vi "DBClient2.vi"() -> ()   [LabVIEW 2015]
uses:
  <vilib>/addons/database/Connection.llb/DB Tools Open Connec (Path).vi
  <vilib>/addons/database/Connection.llb/Conn Execute.vi
  <vilib>/addons/database/Recordset.llb/Rec Fetch Recordset Data (R).vi
  <vilib>/addons/database/Recordset.llb/Rec Destroy - Connection.vi
  <vilib>/addons/database/_DB Variant To Data/Database Variant To Data.xnode
  <vilib>/addons/database/NI_Database_API.lvlib
panel:
  in  "stop":bool
  out "Table link_buku_kategori":string[][](table)
  out "Table link_buku_pengarang":string[][](table)
  out "Table Buku":string[][](table)
  in  "Insert Button link_buku_kategori":bool
  in  "kategori_id lbk":string
  in  "buku_isbn lbk":string
  in  "Insert Button link_buku_pengarang":bool
  in  "pengarang_id lbp":string
  in  "buku_isbn lbp":string
  in  "buku_harga":string
  in  "buku_deskripsi":string
  in  "buku_jmlhalaman":string
  in  "buku_tgl_terbit":string
  in  "penerbit_id buku":string
  in  "buku_judul":string
  in  "buku_ISBN":string
  in  "Insert Button Buku":bool
  out "Table Penerbit":string[][](table)
  in  "Insert Button Penerbit":bool
  in  "Nama Penerbit":string
  in  "ID Penerbit":string
  out "Table Kategori":string[][](table)
  in  "Nama Kategori":string
  in  "ID Kategori":string
  in  "Insert Button Kategori":bool
  in  "Nama Pengarang":string
  in  "ID Pengarang":string
  in  "Insert Button Pengarang":bool
  out "Table Pengarang":string[][](table)
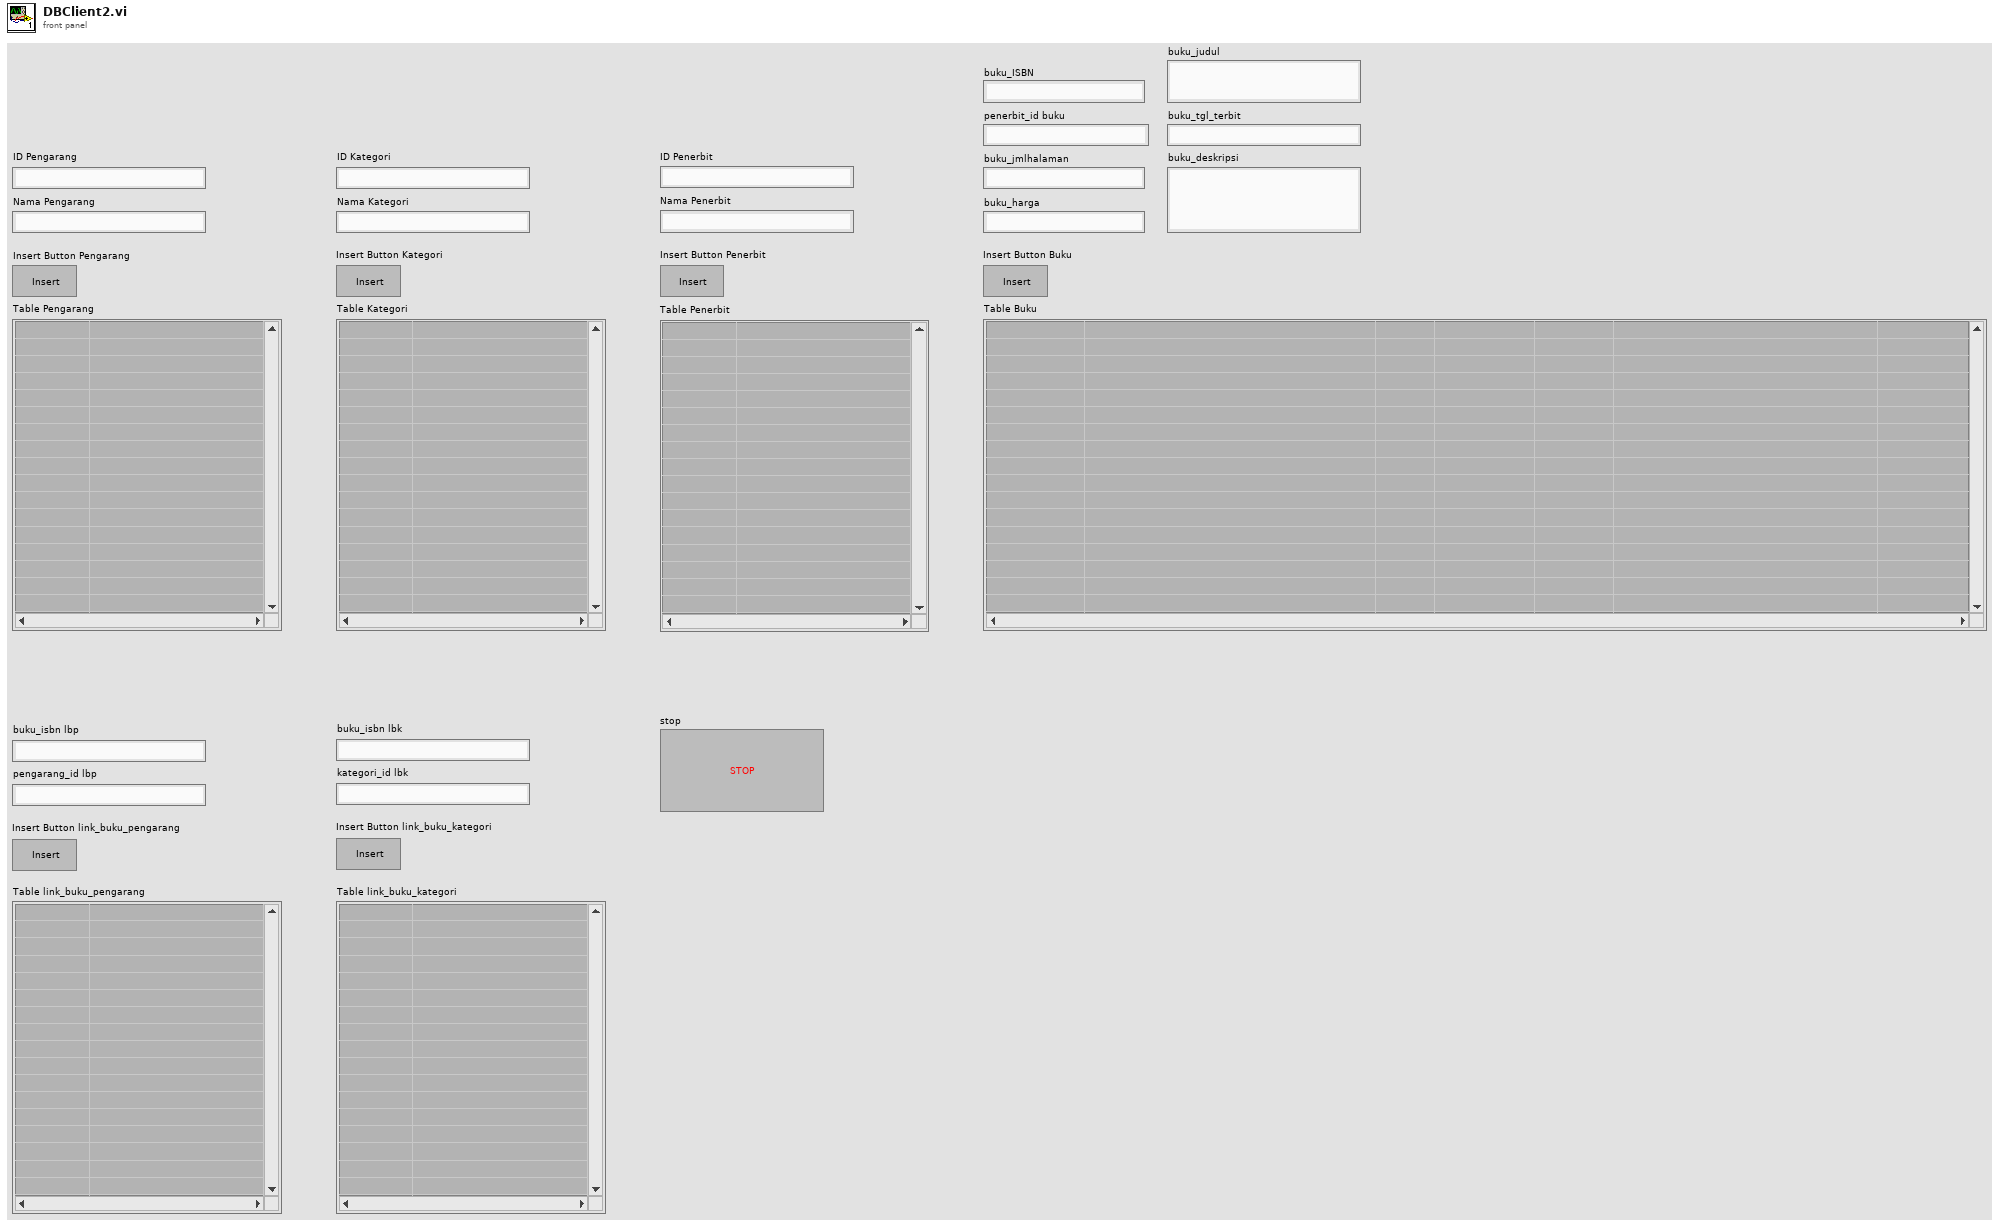
[diagram p1: front panel]
types:
  T1 = typedef "NI_Database_API.lvlib/Conn ObjectReference.ctl" = refnum<k1>
  T2 = typedef "NI_Database_API.lvlib/Rec ObjectReference.ctl" = refnum<k1>
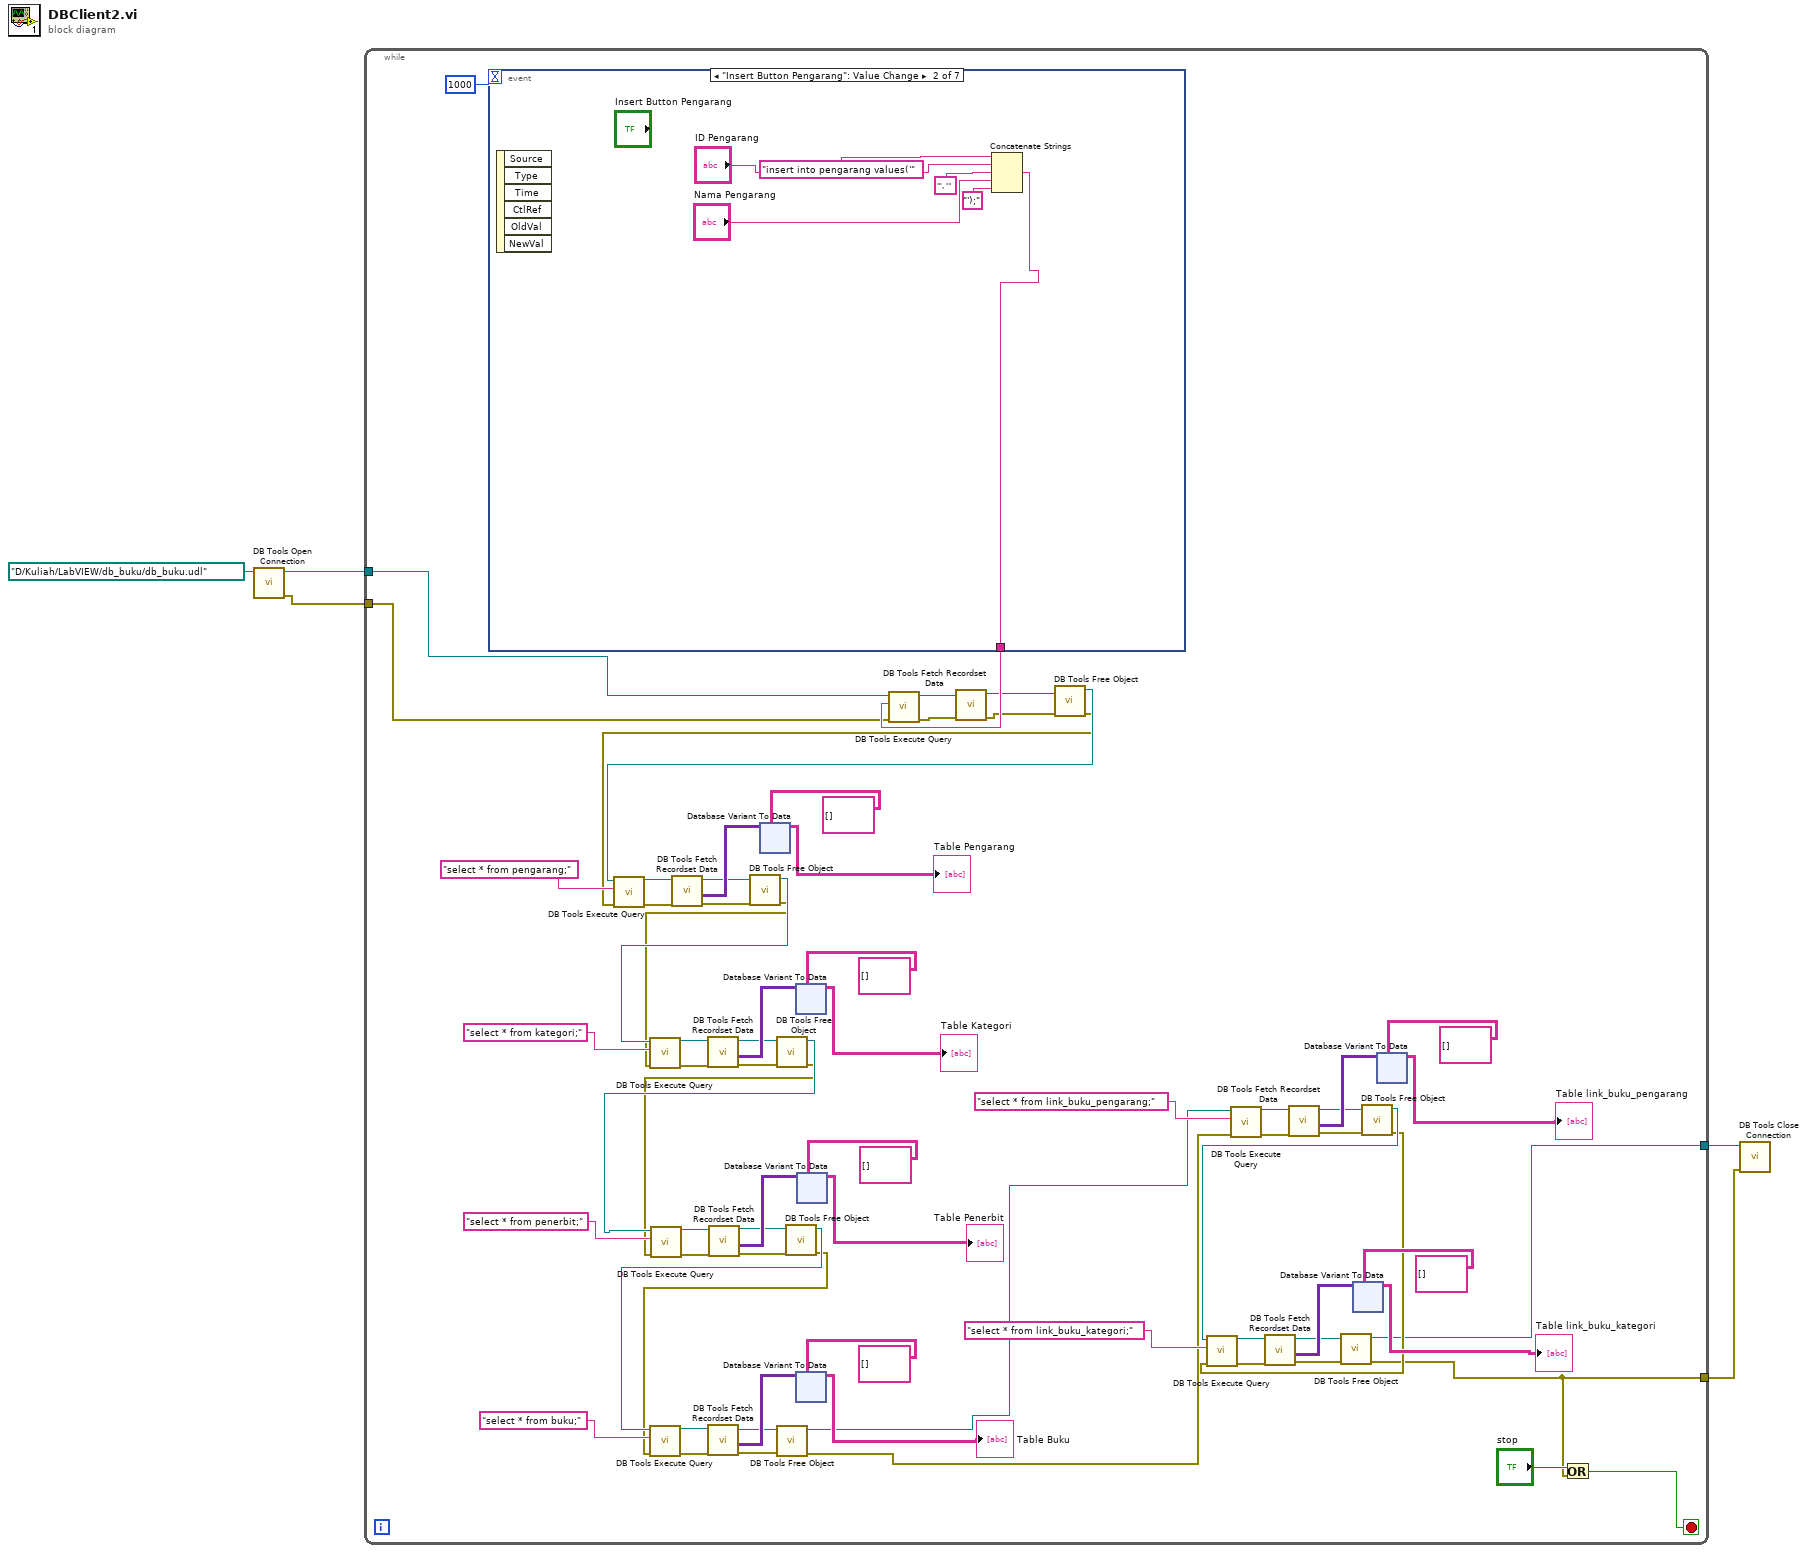
[diagram p0: block diagram]
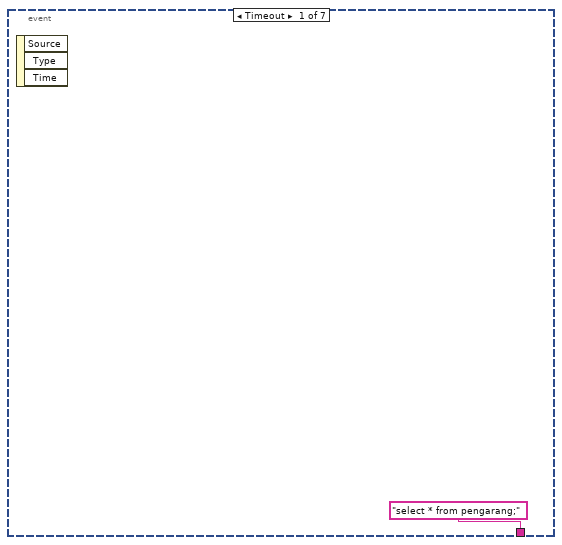
[diagram p2: hidden frame]
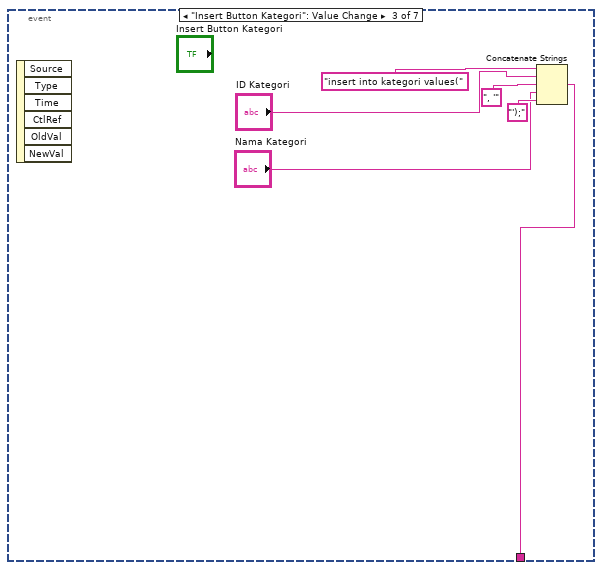
[diagram p3: hidden frame]
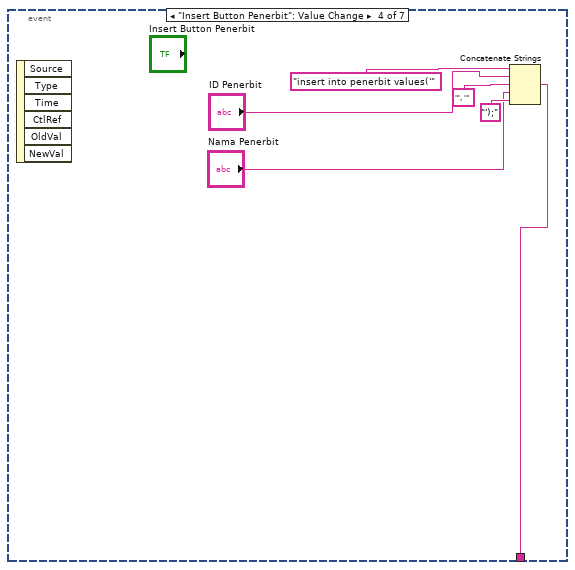
[diagram p4: hidden frame]
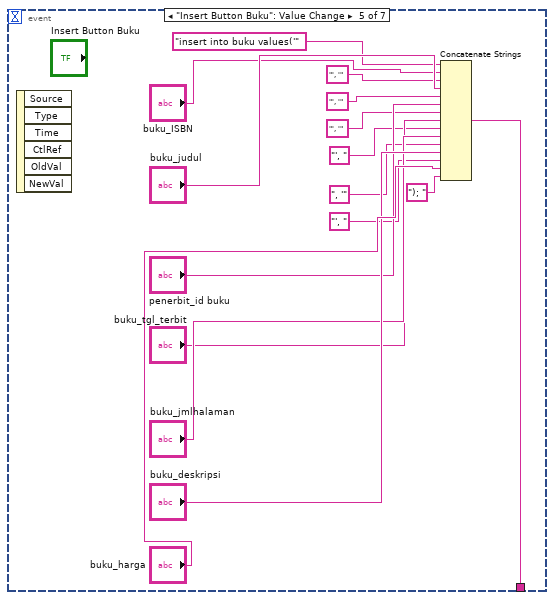
[diagram p5: hidden frame]
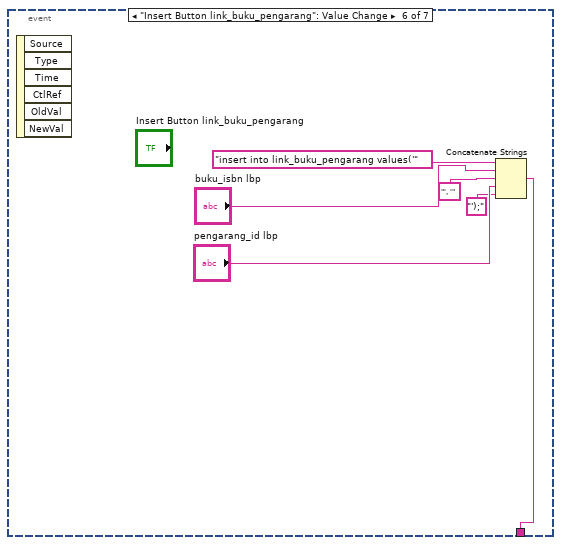
[diagram p6: hidden frame]
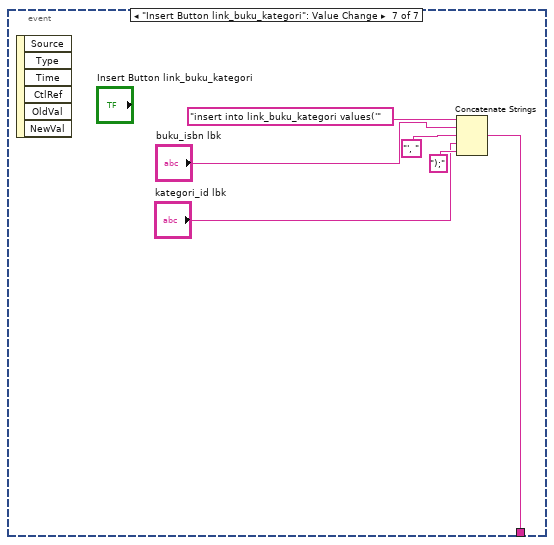
[diagram p7: hidden frame]
diagram:
  n1 = call-poly <vilib>:"DB Tools Open Connection.vi"("connection information"=path "D:/Kuliah/LabVIEW/db_buku/db_buku.udl") -> ("error out"=w4:errorcluster, "connection reference"=w5:T1)  [unwired: 7 in]
  n2 = while {
    tunnel: w5 -> [w38]
    tunnel: w4 -> [w34]
    tunnel: [w9] -> w3
    tunnel: [w6] -> w2
    stop <- w8 stop-if-true
    n3 = event shown="[1] \"Insert Button Pengarang\": Value Change" {
      selector: _ -> [_ _ _ _ _ _ _]
      dyn-events: _ -> [_ _ _ _ _ _ _]
      timeout: 1000 -> [_ _ _ _ _ _ _]
      tunnel: ["select * from pengarang;" w299 w305 w311 w317 w333 w339] -> w70
      event Timeout {
        n4 = event-data() -> ()  [unwired: 1 in, 3 out]
      }
      event "Insert Button Pengarang": Value Change {
        n5 = event-data() -> ()  [unwired: 1 in, 6 out]
        n6 = Concatenate Strings("insert into pengarang values('" ("string"), "ID Pengarang", "', '" ("string"), "Nama Pengarang", "');" ("string")) -> (w299:string)
      }
      event "Insert Button Kategori": Value Change {
        n7 = event-data() -> ()  [unwired: 1 in, 6 out]
        n8 = Concatenate Strings("insert into kategori values(" ("string"), "ID Kategori", ", '" ("string"), "Nama Kategori", "');" ("string")) -> (w305:string)
      }
      event "Insert Button Penerbit": Value Change {
        n9 = event-data() -> ()  [unwired: 1 in, 6 out]
        n10 = Concatenate Strings("insert into penerbit values('" ("string"), "ID Penerbit", "', '" ("string"), "Nama Penerbit", "');" ("string")) -> (w311:string)
      }
      event "Insert Button Buku": Value Change {
        n11 = event-data() -> ()  [unwired: 1 in, 6 out]
        n12 = Concatenate Strings("insert into buku values('" ("string"), "buku_ISBN", "', '" ("string"), "buku_judul", "', '" ("string"), "penerbit_id buku", "', '" ("string"), "buku_tgl_terbit", "', " ("string"), "buku_jmlhalaman", ", '" ("string"), "buku_deskripsi", "', " ("string"), "buku_harga", "); " ("string")) -> (w317:string)
      }
      event "Insert Button link_buku_pengarang": Value Change {
        n13 = event-data() -> ()  [unwired: 1 in, 6 out]
        n14 = Concatenate Strings("insert into link_buku_pengarang values('" ("string"), "buku_isbn lbp", "', '" ("string"), "pengarang_id lbp", "');" ("string")) -> (w333:string)
      }
      event "Insert Button link_buku_kategori": Value Change {
        n15 = event-data() -> ()  [unwired: 1 in, 6 out]
        n16 = Concatenate Strings("insert into link_buku_kategori values('" ("string"), "buku_isbn lbk", "', " ("string"), "kategori_id lbk", ");" ("string")) -> (w339:string)
      }
    }
    n17 = call-poly <vilib>:"DB Tools Execute Query.vi"("error in (no error)"=w34, "SQL query"=w70, "connection reference"=w38) -> ("error out"=w77:errorcluster, "recordset reference"=w68:T2)  [unwired: 5 in]
    n18 = call-poly <vilib>:"DB Tools Fetch Recordset Data.vi"("error in (no error)"=w77, "recordset reference"=w68) -> ("error out"=w33:errorcluster, "recordset reference out"=w36:T2)  [unwired: 3 in, 1 out]
    n19 = call-poly <vilib>:"DB Tools Free Object.vi"("error in (no error)"=w33, "recordset reference"=w36) -> ("error out"=w14:errorcluster, "connection reference"=w21:T1)  [unwired: 8 in]
    n20 = call-poly <vilib>:"DB Tools Execute Query.vi"("error in (no error)"=w14, "SQL query"="select * from pengarang;" ("string"), "connection reference"=w21) -> ("error out"=w75:errorcluster, "recordset reference"=w76:T2)  [unwired: 5 in]
    n21 = call-poly <vilib>:"DB Tools Fetch Recordset Data.vi"("error in (no error)"=w75, "recordset reference"=w76) -> ("error out"=w32:errorcluster, "recordset data"=w73:variant[][], "recordset reference out"=w35:T2)  [unwired: 3 in]
    n22 = call-poly <vilib>:"DB Tools Free Object.vi"("error in (no error)"=w32, "recordset reference"=w35) -> ("error out"=w15:errorcluster, "connection reference"=w20:T1)  [unwired: 8 in]
    n23 = call-poly <vilib>:"DB Tools Execute Query.vi"("error in (no error)"=w15, "SQL query"="select * from kategori;" ("string"), "connection reference"=w20) -> ("error out"=w66:errorcluster, "recordset reference"=w67:T2)  [unwired: 5 in]
    n24 = call-poly <vilib>:"DB Tools Fetch Recordset Data.vi"("error in (no error)"=w66, "recordset reference"=w67) -> ("error out"=w30:errorcluster, "recordset data"=w64:variant[][], "recordset reference out"=w31:T2)  [unwired: 3 in]
    n25 = xnode "Database Variant To Data"("database variant"=w73, "type"=string[][] []) -> ("data"=→"Table Pengarang":string[][])  [unwired: 1 in, 1 out]
    n26 = call-poly <vilib>:"DB Tools Free Object.vi"("error in (no error)"=w30, "recordset reference"=w31) -> ("error out"=w13:errorcluster, "connection reference"=w19:T1)  [unwired: 8 in]
    n27 = call-poly <vilib>:"DB Tools Execute Query.vi"("error in (no error)"=w13, "SQL query"="select * from penerbit;" ("string"), "connection reference"=w19) -> ("error out"=w60:errorcluster, "recordset reference"=w61:T2)  [unwired: 5 in]
    n28 = call-poly <vilib>:"DB Tools Fetch Recordset Data.vi"("error in (no error)"=w60, "recordset reference"=w61) -> ("error out"=w28:errorcluster, "recordset data"=w58:variant[][], "recordset reference out"=w29:T2)  [unwired: 3 in]
    n29 = call-poly <vilib>:"DB Tools Free Object.vi"("error in (no error)"=w28, "recordset reference"=w29) -> ("error out"=w12:errorcluster, "connection reference"=w18:T1)  [unwired: 8 in]
    n30 = call-poly <vilib>:"DB Tools Execute Query.vi"("error in (no error)"=w12, "SQL query"="select * from buku;" ("string"), "connection reference"=w18) -> ("error out"=w54:errorcluster, "recordset reference"=w55:T2)  [unwired: 5 in]
    n31 = call-poly <vilib>:"DB Tools Fetch Recordset Data.vi"("error in (no error)"=w54, "recordset reference"=w55) -> ("error out"=w26:errorcluster, "recordset data"=w52:variant[][], "recordset reference out"=w27:T2)  [unwired: 3 in]
    n32 = call-poly <vilib>:"DB Tools Free Object.vi"("error in (no error)"=w26, "recordset reference"=w27) -> ("error out"=w11:errorcluster, "connection reference"=w17:T1)  [unwired: 8 in]
    n33 = xnode "Database Variant To Data"("database variant"=w64, "type"=string[][] []) -> ("data"=→"Table Kategori":string[][])  [unwired: 1 in, 1 out]
    n34 = xnode "Database Variant To Data"("database variant"=w52, "type"=string[][] []) -> ("data"=→"Table Buku":string[][])  [unwired: 1 in, 1 out]
    n35 = xnode "Database Variant To Data"("database variant"=w58, "type"=string[][] []) -> ("data"=→"Table Penerbit":string[][])  [unwired: 1 in, 1 out]
    n36 = call-poly <vilib>:"DB Tools Execute Query.vi"("error in (no error)"=w11, "SQL query"="select * from link_buku_pengarang;" ("string"), "connection reference"=w17) -> ("error out"=w48:errorcluster, "recordset reference"=w49:T2)  [unwired: 5 in]
    n37 = call-poly <vilib>:"DB Tools Fetch Recordset Data.vi"("error in (no error)"=w48, "recordset reference"=w49) -> ("error out"=w24:errorcluster, "recordset data"=w46:variant[][], "recordset reference out"=w25:T2)  [unwired: 3 in]
    n38 = call-poly <vilib>:"DB Tools Free Object.vi"("error in (no error)"=w24, "recordset reference"=w25) -> ("error out"=w10:errorcluster, "connection reference"=w16:T1)  [unwired: 8 in]
    n39 = call-poly <vilib>:"DB Tools Execute Query.vi"("error in (no error)"=w10, "SQL query"="select * from link_buku_kategori;" ("string"), "connection reference"=w16) -> ("error out"=w42:errorcluster, "recordset reference"=w43:T2)  [unwired: 5 in]
    n40 = call-poly <vilib>:"DB Tools Fetch Recordset Data.vi"("error in (no error)"=w42, "recordset reference"=w43) -> ("error out"=w22:errorcluster, "recordset data"=w40:variant[][], "recordset reference out"=w23:T2)  [unwired: 3 in]
    n41 = call-poly <vilib>:"DB Tools Free Object.vi"("error in (no error)"=w22, "recordset reference"=w23) -> ("error out"=w6:errorcluster, "connection reference"=w9:T1)  [unwired: 8 in]
    n42 = xnode "Database Variant To Data"("database variant"=w40, "type"=string[][] []) -> ("data"=→"Table link_buku_kategori":string[][])  [unwired: 1 in, 1 out]
    n43 = xnode "Database Variant To Data"("database variant"=w46, "type"=string[][] []) -> ("data"=→"Table link_buku_pengarang":string[][])  [unwired: 1 in, 1 out]
    n44 = Or(x="stop", y=w6) -> (x .or. y?=w8:bool)
  }
  n45 = call <vilib>:"DB Tools Close Connection.vi"("error in (no error)"=w2, "connection reference"=w3) -> ()  [unwired: 5 in, 1 out]
